vi "PSVCH_Formula Edit.vi"(8 "Error In (no error)":errorcluster, 9 "Symbol Path":path, 10 "DAQ2ANA":T2[](array[typedef])=[{"Card Name"="9: NI PXIe-4300 \"PXI1Slot9\"", "Channels Tag"=["PXI1Slot9/ai0", "PXI1Slot9/ai1", "PXI1Slot9/ai2", "PXI1Slot9/ai3", "PXI1Slot9/ai4", "PXI1Slot9/ai5", "PXI1Slot9/ai6", "PXI1Slot9/ai7"], "Channels Name"=["", "", "", "", "", "", "", ""], "Unit"=[]}], 11 "Formula In":string) -> (0 "Error Out":errorcluster, 2 "Formula":string, 3 "Cancel?":bool)   [LabVIEW 2016]
uses:
  Private/Ctrls/PSVCH_All Channels.ctl
  <vilib>/Utility/error.llb/DialogType.ctl
  <vilib>/express/express arith-compare/Formula/XNode/ExpressFormulaBlockNode.xnode
panel:
  in  "Data Source":string(tree)
  in  "Formula":string caption="信号处理"
  out "Error":string caption="错误信息"
  in  "Calculator":T1 caption="计算器"
  in  "Cancel":bool
  in  "OK":bool
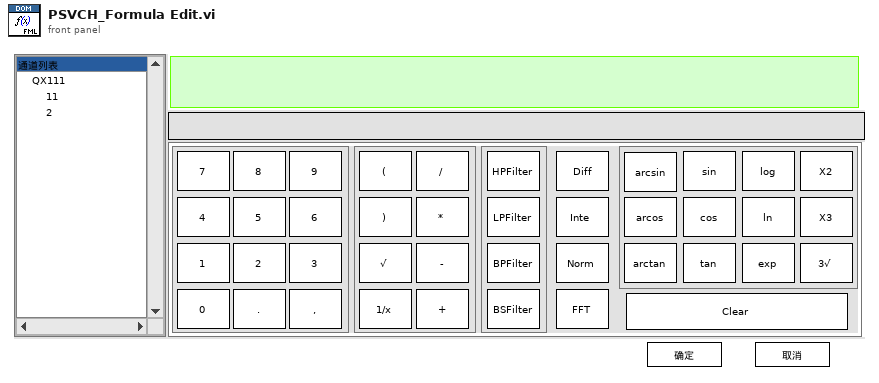
[diagram p1: front panel]
types:
  T1 = cluster{"Cal_0":bool, "Cal_1":bool, "Cal_2":bool, "Cal_3":bool, "Cal_4":bool, "Cal_5":bool, "Cal_6":bool, "Cal_7":bool, "Cal_8":bool, "Cal_9":bool, "Cal_+":bool, "Cal_-":bool, "Cal_*":bool, "Cal_/":bool, "Cal_sin":bool, "Cal_cos":bool, "Cal_diff":bool, "Cal_inte":bool, "Cal_Clear":bool, "Cal_.":bool, "Cal_(":bool, "Cal_)":bool, "Cal_fft":bool, "Cal_,":bool, "Cal_BSFilter":bool, "Cal_BPFilter":bool, "Cal_LPFilter":bool, "Cal_Reciprocal":bool, "Cal_HPFilter":bool, "Cal_Normalize":bool, "Cal_√":bool, "Cal_sinh":bool, "Cal_cosh":bool, "Cal_tan":bool, "Cal_Tanh":bool, "Cal_log":bool, "Cal_ln":bool, "Cal_exp":bool, "Cal_X2":bool, "Cal_X3":bool, "Cal_3√":bool}
  T2 = typedef "PSVCH_All Channels.ctl" = cluster{"Card Name":string, "Channels Tag":string[], "Channels Name":string[], "Unit":string[]}
  T3 = cluster{"VarTag[]":string[], "VarTag[] 2":string[], "Type":variant[]}
  T4 = cluster{"Error":errorcluster, "Exit":bool, "Cancel?":bool, "Ref":cluster{"Formula":refnum<vi>, "OK":refnum<vi>, "Error":refnum<vi>, "Data Source":refnum<vi>}, "Formula":string, "DAQ2ANA":T2[], "VarList":cluster{"Tag":string[], "Name":string[], "Type":variant[]}, "Symbol Path":path}
  T5 = enum8{"Enabled", "Disabled", "Disabled and Grayed Out"}
  T6 = typedef "LVPoint32TypeDef.ctl" = cluster{"Horizontal":i32, "Vertical":i32}
  T7 = cluster{"data name":string, "drag data":variant}[]
  T8 = cluster{"TREE PNG":path, "User Guide":path, "DefaultSave":path, "BuildPath":path, "Image":path, "Modules":path, "Configuration":path, "License":path, "SplitFiles":path, "System.ini":path}
  T9 = cluster{"Tag":string[], "Name":string[], "Type":variant[]}
  T10 = typedef "DialogType.ctl" = u16
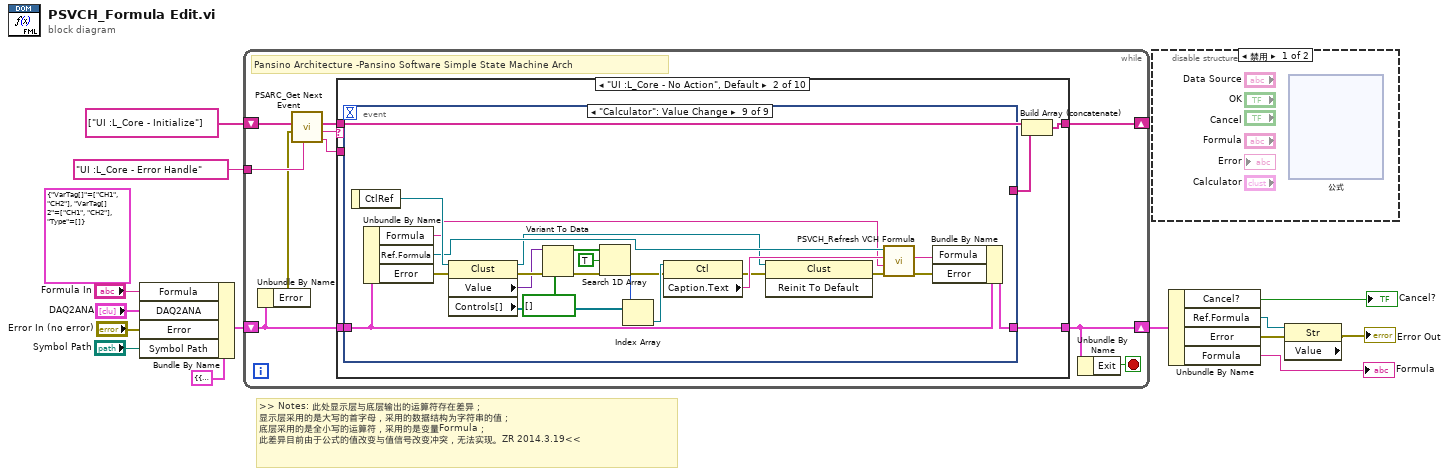
[diagram p0: block diagram]
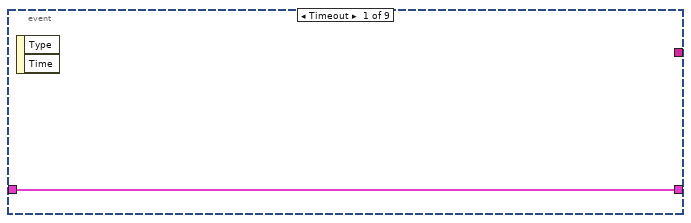
[diagram p3: hidden frame]
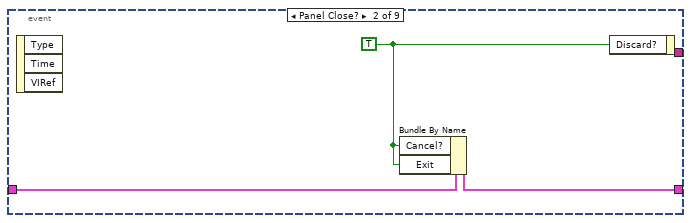
[diagram p4: hidden frame]
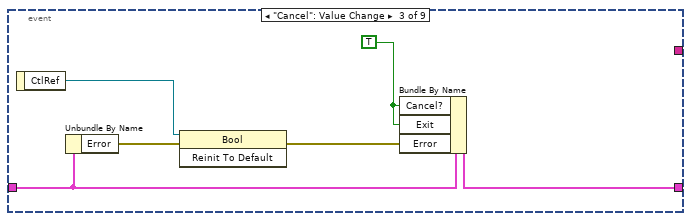
[diagram p5: hidden frame]
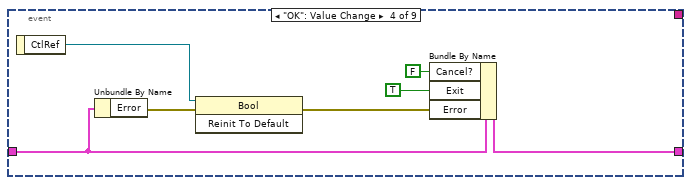
[diagram p6: hidden frame]
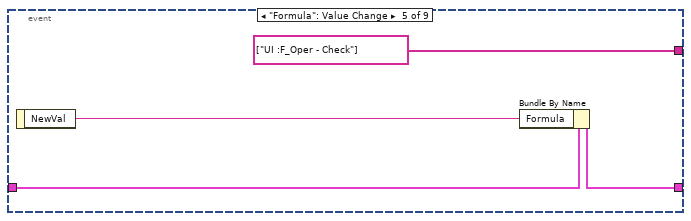
[diagram p7: hidden frame]
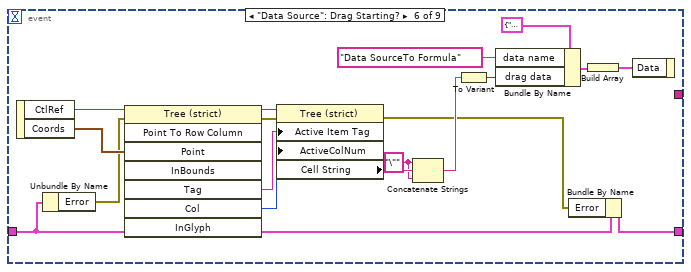
[diagram p8: hidden frame]
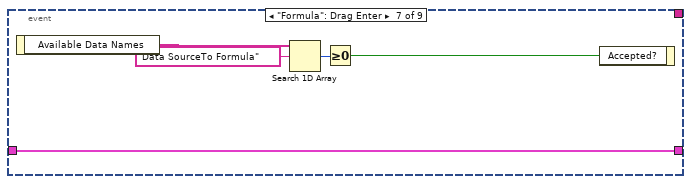
[diagram p9: hidden frame]
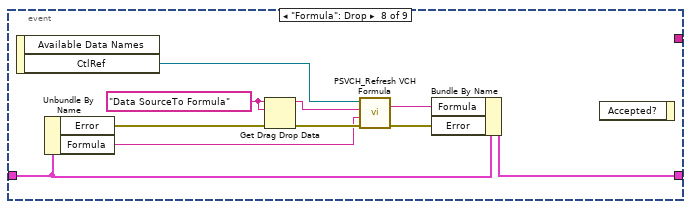
[diagram p10: hidden frame]
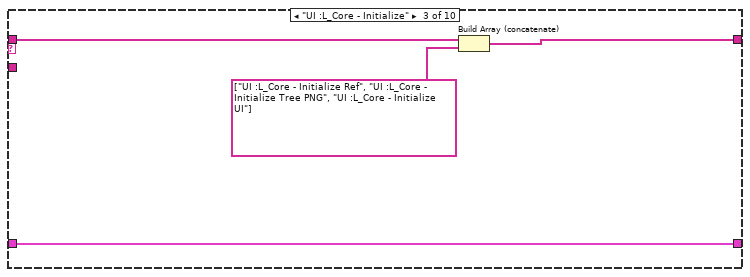
[diagram p11: hidden frame]
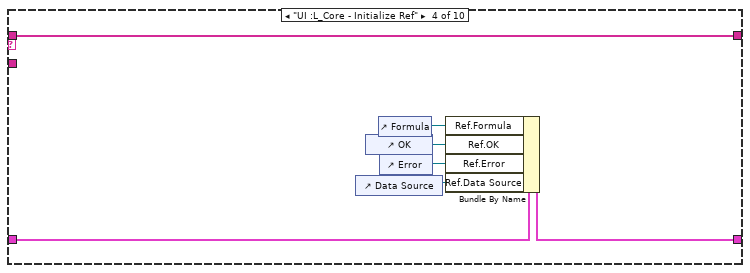
[diagram p12: hidden frame]
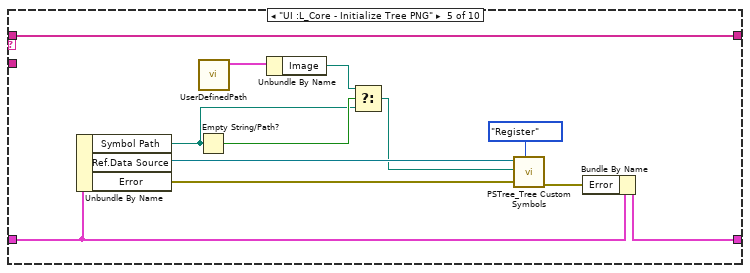
[diagram p13: hidden frame]
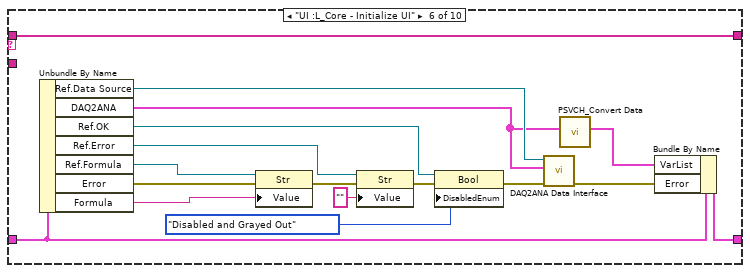
[diagram p14: hidden frame]
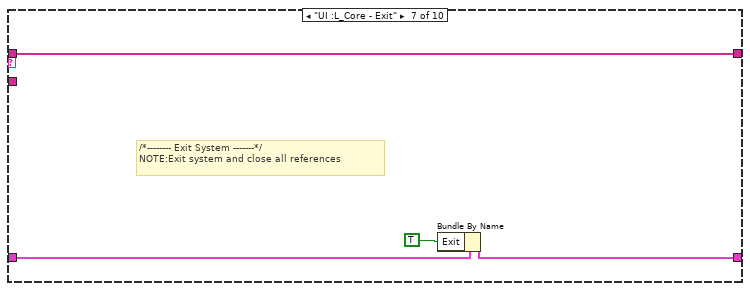
[diagram p15: hidden frame]
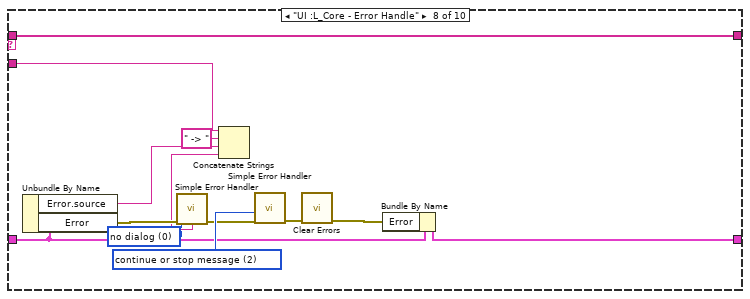
[diagram p16: hidden frame]
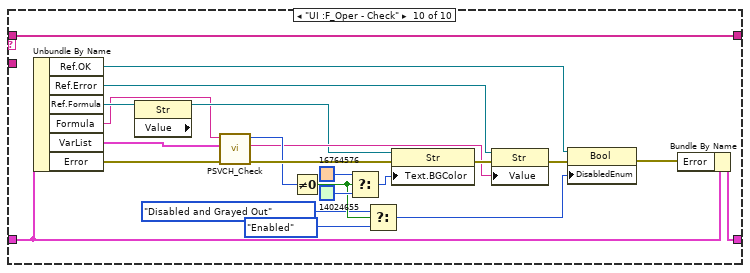
[diagram p18: hidden frame]
diagram:
  (unwired) T3 {"VarTag[]"=["CH1", "CH2"], "VarTag[] 2"=["CH1", "CH2"], "Type"=[]} ("VarList")
  # ">> Notes: 此处显示层与底层输出的运算符存在差异；\n显示层采用的是大写的首字母，采用的数据结构为字符串的值；\n底层采用的是全小写的运算符，采用的是变量Formula；\n此差异目前由于公式的值改变与值信号改变冲突，无法实现。ZR 2014.3.19<<"
  n1 = Bundle By Name(cluster=T4 {"Error"={"status"=FALSE, "code"=0, "source"=""}, "Exit"=FALSE, "Cancel?"=FALSE, "Ref"={"Formula"=refnum, "OK"=refnum, "Error"=refnum, "Data Source"=refnum}, "Formula"="", "DAQ2ANA"=[], "VarList"={"Tag"=[], "Name"=[], "Type"=[]}, "Symbol Path"=path ""} ("Temp Variable"), "Formula"="Formula In", "DAQ2ANA"="DAQ2ANA", "Error"="Error In (no error)", "Symbol Path"="Symbol Path") -> (w7:T4)
  n2 = while {
    tunnel: "UI :L_Core - Error Handle" ("Error Handle") -> [w23]
    shift-right: [w21] -> _
    shift-left: string[] ["UI :L_Core - Initialize"] -> [w24]
    shift-right: [w18] -> w11
    shift-left: w7 -> [w20]
    stop <- w17 stop-if-true
    # "Pansino Architecture -Pansino Software Simple State Machine Arch"
    n3 = Unbundle By Name(w20) -> ("Error"=w19:errorcluster)
    n4 = call <vilib>:"PSARC_Get Next Event.vi"("Error Handle"=w23, "error in (no error)"=w19, "event queue in"=w24) -> ("prev event"=w15:string, "next event"=w16:string, "event queue out"=w22:string[])  [unwired: 3 in]
    n5 = case shown="\"UI :L_Core - No Action\", Default" w16 {
      tunnel: w22 -> [w26 w31 w110 w117 w129 w146 w150 w163 w165 w188]
      tunnel: [w26 w30 w108 w117 w129 w146 w150 w163 w165 w188] -> w21
      tunnel: w20 -> [w25 w29 w109 w116 w126 w145 w149 w160 w164 w187]
      tunnel: [w25 w28 w109 w115 w124 w140 w148 w159 w164 w186] -> w18
      tunnel: w15 -> [_ _ _ _ _ _ _ w152 _ _]
      frame "----------Core Status----------" {
      }
      frame "UI :L_Core - No Action", Default {
        n6 = event shown="[8] \"Calculator\": Value Change" {
          selector: _ -> [_ _ _ _ _ _ _ _ _]
          dyn-events: _ -> [_ _ _ _ _ _ _ _ _]
          timeout: _ -> [_ _ _ _ _ _ _ _ _]
          tunnel: w29 -> [w32 w35 w38 w43 w52 w68 w72 w85 w106]
          tunnel: [w32 w34 w41 w48 w50 w61 w72 w81 w105] -> w28
          tunnel: [_ _ _ _ string[] ["UI :F_Oper - Check"] ("数组") _ _ _ _] -> w27
          event Timeout {
            n7 = event-data() -> ()  [unwired: 1 in, 2 out]
          }
          event Panel Close? {
            w33 = TRUE ("放弃？")
            n8 = event-data() -> ()  [unwired: 1 in, 3 out]
            n9 = Bundle By Name(cluster=w35, "Cancel?"=w33, "Exit"=w33) -> (w34:T4)
            n10 = event-data("Discard?"=w33) -> ()  [unwired: 1 in, 1 out]
          }
          event "Cancel": Value Change {
            w40 = TRUE ("放弃？")
            n11 = event-data() -> ("CtlRef"=w36:refnum<vi>)  [unwired: 1 in]
            n12 = Unbundle By Name(w38) -> ("Error"=w37:errorcluster)
            n13 = invoke class="Bool" method="Reinit To Default"(reference=w36, error in=w37) -> (error out=w39:errorcluster)  [unwired: 1 in, 2 out]
            n14 = Bundle By Name(cluster=w38, "Cancel?"=w40, "Exit"=w40, "Error"=w39) -> (w41:T4)
          }
          event "OK": Value Change {
            n15 = event-data() -> ("CtlRef"=w44:refnum<vi>)  [unwired: 1 in]
            n16 = Unbundle By Name(w43) -> ("Error"=w42:errorcluster)
            n17 = invoke class="Bool" method="Reinit To Default"(reference=w44, error in=w42) -> (error out=w45:errorcluster)  [unwired: 1 in, 2 out]
            n18 = Bundle By Name(cluster=w43, "Cancel?"=FALSE, "Exit"=TRUE, "Error"=w45) -> (w48:T4)
          }
          event "Formula": Value Change {
            n19 = event-data() -> ("NewVal"=w49:string)  [unwired: 1 in]
            n20 = Bundle By Name(cluster=w52, "Formula"=w49) -> (w50:T4)
          }
          event "Data Source": Drag Starting? {
            w55 = "\"" ("字符串")
            n21 = event-data() -> ("CtlRef"=w70:refnum<vi>, "Coords"=w69:T6)  [unwired: 1 in]
            n22 = Unbundle By Name(w68) -> ("Error"=w67:errorcluster)
            n23 = invoke class="Tree (strict)" method="Point To Row Column"(reference=w70, error in=w67, "Point"=w69) -> (reference out=w60:refnum<vi>, error out=w59:errorcluster, "Tag"=w58:string, "Col"=w57:i32)  [unwired: 5 in, 4 out]
            n24 = property class="Tree (strict)"(reference=w60, error in=w59, "Active Item Tag"=w58, "ActiveColNum"=w57) -> (error out=w53:errorcluster, "Cell String"=w56:string)  [unwired: 1 out]
            n25 = Concatenate Strings(w55, w56, w55) -> (w54:string)
            n26 = To Variant(anything=w54) -> (Variant=w64:variant)
            n27 = Bundle By Name(cluster=cluster{"data name":string, "drag data":variant} {"data name"="", "drag data"=variant}, "data name"="Data SourceTo Formula" ("元素"), "drag data"=w64) -> (w63:cluster{"data name":string, "drag data":variant})
            n28 = Bundle By Name(cluster=w68, "Error"=w53) -> (w61:T4)
            n29 = Build Array(w63) -> (w62:T7)
            n30 = event-data("Data"=w62) -> ()  [unwired: 1 in, 1 out]
          }
          event "Formula": Drag Enter {
            n31 = event-data() -> ("Available Data Names"=w74:string[])  [unwired: 1 in]
            n32 = Search 1D Array(1D array=w74, element="Data SourceTo Formula" ("元素")) -> (index of element=w75:i32)  [unwired: 1 in]
            n33 = Greater Or Equal To 0?(x=w75) -> (x >= 0?=w73:bool)
            n34 = event-data("Accepted?"=w73) -> ()  [unwired: 1 in, 1 out]
          }
          event "Formula": Drop {
            w83 = "Data SourceTo Formula" ("元素")
            n35 = event-data() -> ("CtlRef"=w78:refnum<vi>)  [unwired: 1 in, 1 out]
            n36 = Unbundle By Name(w85) -> ("Error"=w84:errorcluster, "Formula"=w76:string)
            n37 = Get Drag Drop Data(6:w84, 8:w83, 9:w83) -> (0:w82:errorcluster, 3:w79:string)
            n38 = call "PSVCH_Refresh VCH Formula.vi"("error in"=w82, "Formula In"=w76, "String"=w79, "VCH_Formula"=w78) -> ("error out"=w80:errorcluster, "result string"=w77:string)  [unwired: 6 in]
            n39 = Bundle By Name(cluster=w85, "Formula"=w77, "Error"=w80) -> (w81:T4)
            n40 = event-data() -> ()  [unwired: 2 in, 1 out]
          }
          event "Calculator": Value Change {
            n41 = event-data() -> ("CtlRef"=w94:refnum<vi>)  [unwired: 1 in]
            n42 = Unbundle By Name(w106) -> ("Formula"=w86:string, "Ref.Formula"=w91:refnum<vi>, "Error"=w93:errorcluster)
            n43 = property class="Clust"(reference=w94, error in=w93) -> (reference out=w88:refnum<vi>, error out=w96:errorcluster, "Value"=w95:variant, "Controls[]"=w100:refnum<vi>[])
            n44 = Variant To Data(error in=w96, type=bool[] [], Variant=w95) -> (data=w98:bool[], error out=w102:errorcluster)
            n45 = Search 1D Array(1D array=w98, element=TRUE ("元素")) -> (index of element=w101:i32)  [unwired: 1 in]
            n46 = Index Array(array=w100, index=w101) -> (element=w103:refnum<vi>)
            n47 = property class="Ctl"(reference=w103, error in=w102) -> (error out=w90:errorcluster, "Caption.Text"=w92:string)  [unwired: 1 out]
            n48 = invoke class="Clust" method="Reinit To Default"(reference=w88, error in=w90) -> (error out=w89:errorcluster)  [unwired: 1 in, 2 out]
            n49 = call "PSVCH_Refresh VCH Formula.vi"("error in"=w89, "Formula In"=w86, "String"=w92, "VCH_Formula"=w91) -> ("error out"=w104:errorcluster, "result string"=w87:string)  [unwired: 6 in]
            n50 = Bundle By Name(cluster=w106, "Formula"=w87, "Error"=w104) -> (w105:T4)
          }
        }
        n51 = Build Array (concatenate)(w31, w27) -> (w30:string[])
      }
      frame "UI :L_Core - Initialize" {
        n52 = Build Array (concatenate)(w110, string[] ["UI :L_Core - Initialize Ref", "UI :L_Core - Initialize Tree PNG", "UI :L_Core - Initialize UI"] ("数组")) -> (w108:string[])
      }
      frame "UI :L_Core - Initialize Ref" {
        n53 = control-ref of="Data Source"() -> (w111:refnum<vi>)
        n54 = control-ref of="OK"() -> (w113:refnum<vi>)
        n55 = control-ref of="Formula"() -> (w114:refnum<vi>)
        n56 = control-ref of="Error"() -> (w112:refnum<vi>)
        n57 = Bundle By Name(cluster=w116, "Ref.Formula"=w114, "Ref.OK"=w113, "Ref.Error"=w112, "Ref.Data Source"=w111) -> (w115:T4)
      }
      frame "UI :L_Core - Initialize Tree PNG" {
        n58 = Unbundle By Name(w126) -> ("Symbol Path"=w121:path, "Ref.Data Source"=w127:refnum<vi>, "Error"=w128:errorcluster)
        n59 = Empty String/Path?(string/path=w121) -> (empty?=w122:bool)
        n60 = call "UserDefinedPath.vi"() -> ("UserDefinedPath"=w118:T8)  [unwired: 11 in]
        n61 = Unbundle By Name(w118) -> ("Image"=w120:path)
        n62 = Select(t=w120, s=w122, f=w121) -> (s? t:f=w119:path)
        n63 = call "PSTree_Tree Custom Symbols.vi"("Operation"=enum16{"Register", "GetIndex"}."Register", "error in (no error)"=w128, "Files"=w119, "tree refnum"=w127) -> ("error out"=w125:errorcluster)  [unwired: 6 in, 1 out]
        n64 = Bundle By Name(cluster=w126, "Error"=w125) -> (w124:T4)
      }
      frame "UI :L_Core - Initialize UI" {
        n65 = Unbundle By Name(w145) -> ("Ref.Data Source"=w136:refnum<vi>, "DAQ2ANA"=w135:T2[], "Ref.OK"=w142:refnum<vi>, "Ref.Error"=w131:refnum<vi>, "Ref.Formula"=w144:refnum<vi>, "Error"=w143:errorcluster, "Formula"=w139:string)
        n66 = property class="Str"(reference=w144, error in=w143, "Value"=w139) -> (error out=w133:errorcluster)  [unwired: 1 out]
        n67 = property class="Str"(reference=w131, error in=w133, "Value"="") -> (error out=w132:errorcluster)  [unwired: 1 out]
        n68 = property class="Bool"(reference=w142, error in=w132, "DisabledEnum"=T5."Disabled and Grayed Out" ("禁用")) -> (error out=w138:errorcluster)  [unwired: 1 out]
        n69 = call "DAQ2ANA Data Interface.vi"("error in (no error)"=w138, "DAQ2ANA"=w135, "Tree Ref"=w136) -> ("error out"=w137:errorcluster)  [unwired: 8 in]
        n70 = call "PSVCH_Convert Data.vi"("DAQ2ANA"=w135) -> ("VarList"=w134:T9)  [unwired: 10 in]
        n71 = Bundle By Name(cluster=w145, "VarList"=w134, "Error"=w137) -> (w140:T4)
      }
      frame "UI :L_Core - Exit" {
        # "/*-------- Exit System -------*/\nNOTE:Exit system and close all references"
        n72 = Bundle By Name(cluster=w149, "Exit"=TRUE) -> (w148:T4)
      }
      frame "UI :L_Core - Error Handle" {
        w151 = T10 0 items=["no dialog", "OK message", "continue or stop message", "OK message + warnings", "continue/stop + warnings"] ("type of dialog (OK msg:1)")
        w162 = T10 2 items=["no dialog", "OK message", "continue or stop message", "OK message + warnings", "continue/stop + warnings"] ("type of dialog (OK msg:1)")
        n73 = Unbundle By Name(w160) -> ("Error.source"=w156:string, "Error"=w157:errorcluster)
        n74 = call <vilib>:"Simple Error Handler.vi"("type of dialog (OK msg:1)"=w151, "error in (no error)"=w157) -> ("error out"=w155:errorcluster, "message"=w154:string)  [unwired: 3 in, 3 out]
        n75 = Concatenate Strings(w152, " -> " ("字符串"), w156, w154) -> ()  [unwired: 1 out]
        n76 = call <vilib>:"Simple Error Handler.vi"("type of dialog (OK msg:1)"=w162, "error in (no error)"=w155) -> ("error out"=w161:errorcluster)  [unwired: 3 in, 4 out]
        n77 = call <vilib>:"Clear Errors.vi"("error in (no error)"=w161) -> ("error out"=w158:errorcluster)  [unwired: 5 in, 1 out]
        n78 = Bundle By Name(cluster=w160, "Error"=w158) -> (w159:T4)
      }
      frame "----------Operation----------" {
      }
      frame "UI :F_Oper - Check" {
        n79 = Unbundle By Name(w187) -> ("Ref.OK"=w176:refnum<vi>, "Ref.Error"=w179:refnum<vi>, "Ref.Formula"=w168:refnum<vi>, "Formula"=w166:string, "VarList"=w170:T9, "Error"=w169:errorcluster)
        n80 = property class="Str" props=["Value"](reference=w168) -> (reference out=w167:refnum<vi>)  [unwired: 1 in, 2 out]
        n81 = call "PSVCH_Check.vi"("Error In (no error)"=w169, "VarList"=w170, "Formula"=w166) -> ("Error Out"=w182:errorcluster, "source"=w178:string, "code"=w181:i32)  [unwired: 6 in]
        n82 = Not Equal To 0?(x=w181) -> (x != 0?=w173:bool)
        n83 = Select(t=u32 16764576 ("Color 2"), s=w173, f=u32 14024655 ("Color")) -> (s? t:f=w183:u32)
        n84 = Select(t=T5."Disabled and Grayed Out", s=w173, f=T5."Enabled" ("禁用")) -> (s? t:f=w171:T5)
        n85 = property class="Str"(reference=w167, error in=w182, "Text.BGColor"=w183) -> (error out=w180:errorcluster)  [unwired: 1 out]
        n86 = property class="Str"(reference=w179, error in=w180, "Value"=w178) -> (error out=w177:errorcluster)  [unwired: 1 out]
        n87 = property class="Bool"(reference=w176, error in=w177, "DisabledEnum"=w171) -> (error out=w175:errorcluster)  [unwired: 1 out]
        n88 = Bundle By Name(cluster=w187, "Error"=w175) -> (w186:T4)
      }
    }
    n89 = Unbundle By Name(w18) -> ("Exit"=w17:bool)
  }
  n90 = disable-structure shown="禁用" {
    frame Disabled {
      n91 = xnode "公式"() -> ()  [unwired: 2 in, 2 out]
    }
    frame Enabled {
    }
  }
  n92 = Unbundle By Name(w11) -> ("Cancel?"=→"Cancel?":bool, "Ref.Formula"=w9:refnum<vi>, "Error"=w8:errorcluster, "Formula"=→"Formula":string)
  n93 = property class="Str" props=["Value"](reference=w9, error in=w8) -> (error out=→"Error Out":errorcluster)  [unwired: 2 out]
